vi "Append Anything to StdOut.vi"(4 "error in (no error)":errorcluster, 7 "Anything":variant) -> (0 "error out":errorcluster)   [LabVIEW 2015, in "StdOut Operations.lvlib"]
uses:
  StdOut Operations.lvlib
  Data Manipulation/Data Manipulation.lvlib
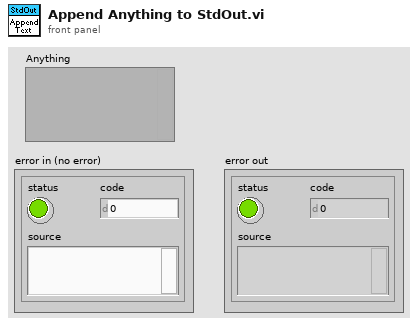
[diagram p1: front panel]
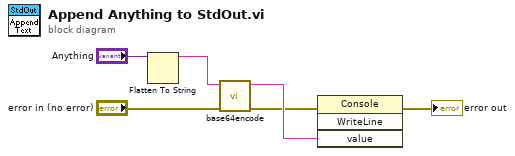
[diagram p0: block diagram]
diagram:
  n1 = Flatten To String(anything="Anything") -> (data string=w4:string)  [unwired: 3 in, 2 out]
  n2 = call "base64encode.vi"("Error In"="error in (no error)", "string in (not encoded)"=w4) -> ("Error Out"=w1:errorcluster, "string out (base64-encoded)"=w2:string)  [unwired: 4 in]
  n3 = invoke class="Console" method="WriteLine"(error in=w1, "value"=w2) -> (error out=→"error out":errorcluster)  [unwired: 2 in, 3 out]
